vi "DashboardHeader.vi"() -> ()   [LabVIEW 2026]
uses:
  DashboardHeader.ctl
panel:
  in  "Cluster":T1
  # "Rozproszone Systemy Pomiarowe - Dashboard LabVIEW"
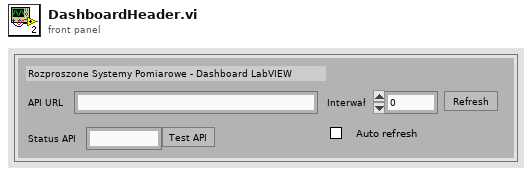
[diagram p1: front panel]
types:
  T1 = typedef "DashboardHeader.ctl" = cluster{"btn_test_api":bool, "refresh":bool, "Auto refresh":bool, "API URL":string, "Interwał":dbl, "Status API":string}
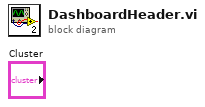
[diagram p0: block diagram]
diagram:
